vi "TestSetLanguage.vi"(8 "error in (no error)":errorcluster) -> (0 "error out":errorcluster)   [LabVIEW 2017]
uses:
  src/Private/RegisterVI.vi
  <vilib>/addons/_JKI Toolkits/Caraya/classes/Test/Test.lvclass
  src/API/JKI Simple Localization.lvlib
  <vilib>/addons/_JKI Toolkits/Caraya/classes/Assert/Assert.lvclass
panel:
  # "See block diagram for unit tests of SetLanguage.vi"
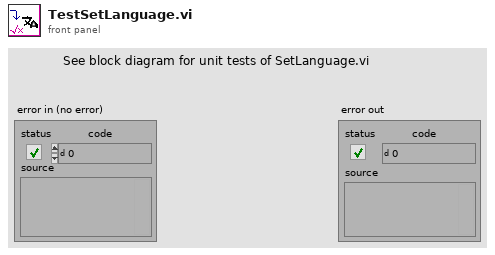
[diagram p1: front panel]
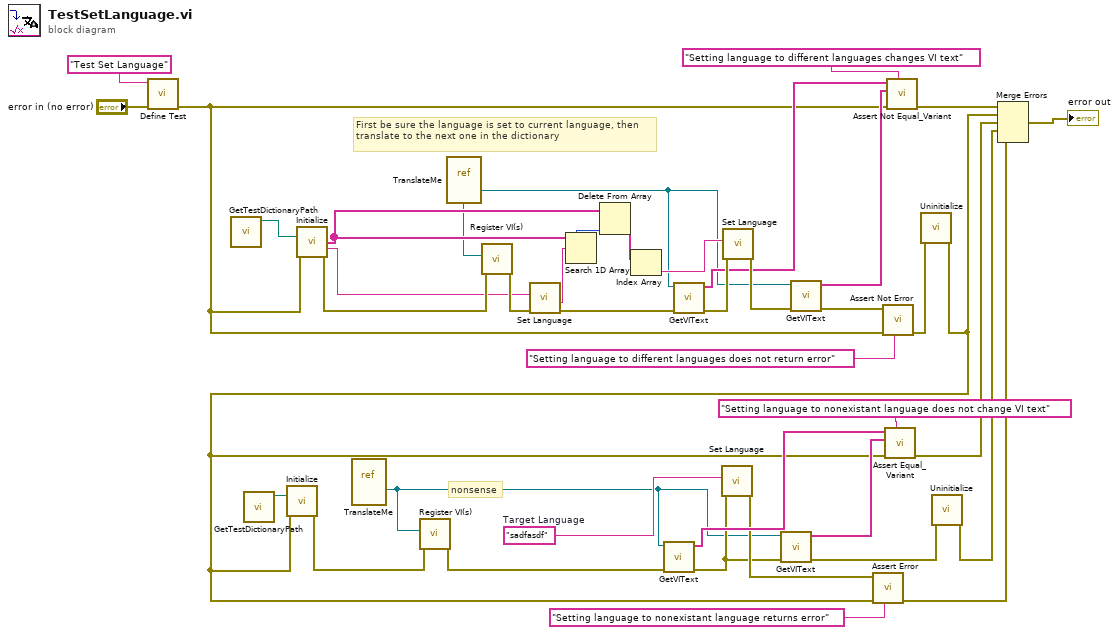
[diagram p0: block diagram]
diagram:
  w26 = "sadfasdf"  # Target Language
  # "nonsense"
  # "First be sure the language is set to current language, then translate to the next one in the dictionary"
  n1 = call <vilib>:"Define Test.vi"("error in (no error)"="error in (no error)", "Label (VI Title)"="Test Set Language") -> ("error out"=w23:errorcluster)  [unwired: 9 in]
  n2 = call "GetTestDictionaryPath.vi"() -> ("Test Dictionary Path"=w38:path)  [unwired: 11 in]
  n3 = call "GetTestDictionaryPath.vi"() -> ("Test Dictionary Path"=w25:path)  [unwired: 11 in]
  n4 = call "Initialize.vi"("Dictionary File Path"=w38, "error in"=w23) -> ("Languages"=w32:string[], "Current Language"=w9:string, "error out"=w15:errorcluster)  [unwired: 10 in, 1 out]
  n5 = vi-ref "TranslateMe.vi"() -> (w8:refnum<vi>)
  n6 = vi-ref "TranslateMe.vi"() -> (w16:refnum<vi>)
  n7 = call-poly "Register VI(s).vi"("error in"=w15, "VI Ref"=w16) -> ("error out"=w14:errorcluster)  [unwired: 8 in, 1 out]
  n8 = call "Set Language.vi"("error in"=w14, "Target Language (current lang)"=w9) -> ("error out"=w10:errorcluster, "Current Language"=w1:string)  [unwired: 8 in]
  n9 = Search 1D Array(1D array=w32, element=w1) -> (index of element=w33:i32)  [unwired: 1 in]
  n10 = Delete From Array(array=w32, index=w33) -> (array with subset deleted=w18:string[])  [unwired: 1 in, 1 out]
  n11 = Index Array(array=w18) -> (element=w17:string)  [unwired: 1 in]
  n12 = call "GetVIText.vi"("error in (no error)"=w10, "VI"=w16) -> ("error out"=w31:errorcluster, "Control Text"=w28:string[])  [unwired: 7 in, 1 out]
  n13 = call "Set Language.vi"("error in"=w31, "Target Language (current lang)"=w17) -> ("error out"=w30:errorcluster)  [unwired: 8 in, 1 out]
  n14 = call "GetVIText.vi"("error in (no error)"=w30, "VI"=w16) -> ("error out"=w29:errorcluster, "Control Text"=w27:string[])  [unwired: 7 in, 1 out]
  n15 = call <vilib>:"Assert Not Error.vi"("Label"="Setting language to different languages does not return error", "error in (no error)"=w23, "Not Error?"=w29) -> ("error out"=w5:errorcluster)  [unwired: 8 in]
  n16 = call <vilib>:"Assert Not Equal_Variant.vi"("Label"="Setting language to different languages changes VI text", "error in (no error)"=w23, "Y"=w27, "X"=w28) -> ("error out"=w36:errorcluster)  [unwired: 7 in]
  n17 = call "Uninitialize.vi"("error in"=w5) -> ("error out"=w4:errorcluster)  [unwired: 10 in]
  n18 = call "Initialize.vi"("Dictionary File Path"=w25, "error in"=w4) -> ("error out"=w7:errorcluster)  [unwired: 10 in, 3 out]
  n19 = call-poly "Register VI(s).vi"("error in"=w7, "VI Ref"=w8) -> ("error out"=w6:errorcluster)  [unwired: 8 in, 1 out]
  n20 = call "GetVIText.vi"("error in (no error)"=w6, "VI"=w8) -> ("error out"=w12:errorcluster, "Control Text"=w21:string[])  [unwired: 7 in, 1 out]
  n21 = call "Set Language.vi"("error in"=w12, "Target Language (current lang)"=w26) -> ("error out"=w13:errorcluster)  [unwired: 8 in, 1 out]
  n22 = call "GetVIText.vi"("error in (no error)"=w12, "VI"=w8) -> ("error out"=w3:errorcluster, "Control Text"=w22:string[])  [unwired: 7 in, 1 out]
  n23 = call <vilib>:"Assert Error.vi"("Label"="Setting language to nonexistant language returns error", "error in (no error)"=w4, "Error?"=w13) -> ("error out"=w11:errorcluster)  [unwired: 8 in]
  n24 = call <vilib>:"Assert Equal_Variant.vi"("Label"="Setting language to nonexistant language does not change VI text", "error in (no error)"=w4, "Y"=w22, "X"=w21) -> ("error out"=w19:errorcluster)  [unwired: 7 in]
  n25 = call "Uninitialize.vi"("error in"=w3) -> ("error out"=w2:errorcluster)  [unwired: 10 in]
  n26 = Merge Errors(w36, w4, w19, w2, w11) -> (→"error out":errorcluster)
